vi "Dragging_Dresser.vi"() -> ()   [LabVIEW 2022 SP3]
panel:
  out "Values of F'":dbl[](array[numeric])
  in  "Mu":dbl
  out "Waveform Graph":dbl[](graph)
  # "Dragging Dresser:\nEnter a value of Mu for the coefficient of kinetic friction.\nThe force per unit weight of the dresser will be populated\ninto the Graph below"
  # "When Mu = 0.1, F' is at a minimum for theta = 6 deg\nWhen Mu = 0.4, F' is at a minimum for theta = 21 deg\nWhen Mu = 1, F' is at a minimum for theta = 44 deg"
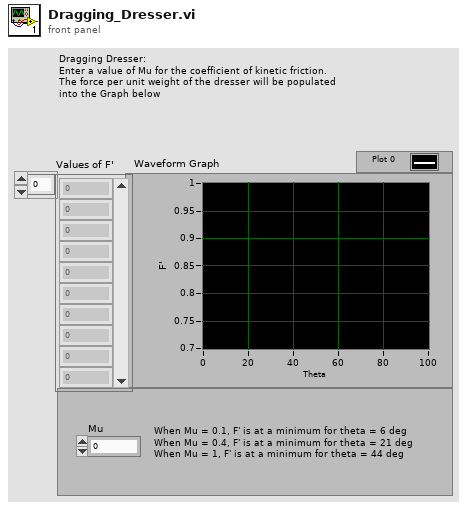
[diagram p1: front panel]
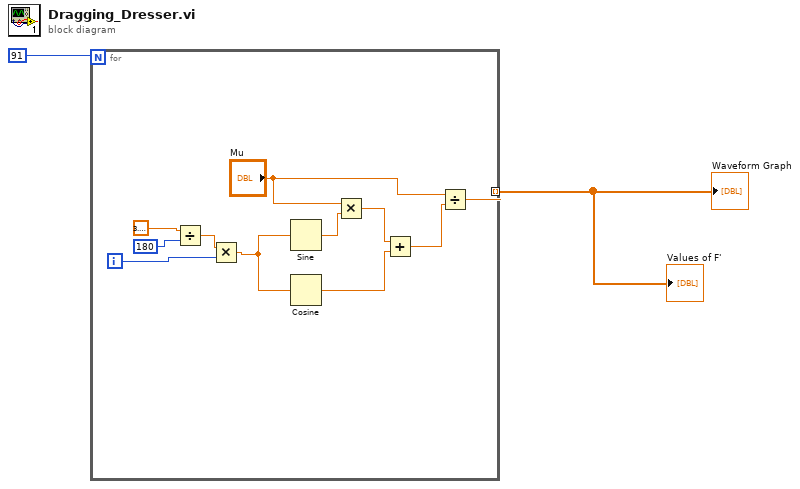
[diagram p0: block diagram]
diagram:
  n1 = for {
    N: 91 -> [_]
    tunnel: [w4] -> w1 mode=indexing
    i -> [w3]
    n2 = Divide(x=3.141592653589793, y=180) -> (x/y=w11:dbl)
    n3 = Multiply(x=w11, y=w3) -> (x*y=w10:dbl)
    n4 = Sine(x=w10) -> (sin(x)=w9:dbl)
    n5 = Cosine(x=w10) -> (cos(x)=w7:dbl)
    n6 = Multiply(x="Mu", y=w9) -> (x*y=w8:dbl)
    n7 = Add(x=w8, y=w7) -> (x+y=w6:dbl)
    n8 = Divide(x="Mu", y=w6) -> (x/y=w4:dbl)
  }
  "Waveform Graph" <- w1
  "Values of F'" <- w1
